vi "niRFUtil FWK Remove All Whitespaces.vi"(7 "Input String":string) -> (8 "Resultant String":string)   [LabVIEW 2015, in "niRFUtil.lvlib"]
uses:
  niRFUtil.lvlib
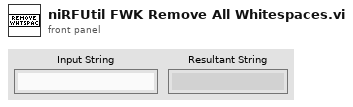
[diagram p1: front panel]
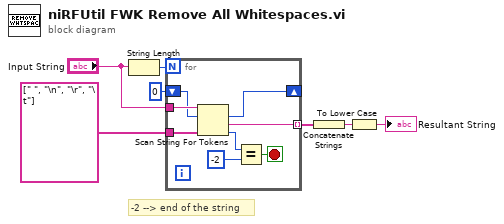
[diagram p0: block diagram]
diagram:
  # "-2 --> end of the string"
  n1 = String Length(string="Input String") -> (length=w7:i32)
  n2 = for {
    N: w7 -> [_]
    tunnel: string[] [" ", "\n", "\r", "\t"] ("Array") -> [w15]
    tunnel: "Input String" -> [w14]
    shift-right: [w8] -> _
    shift-left: 0 -> [w10]
    tunnel: [w9] -> w5 mode=indexing
    stop <- w11 stop-if-true
    n3 = Scan String For Tokens(6:w15, 8:w10, 9:w14) -> (0:w13:i32, 1:w9:string, 2:w8:i32)  [unwired: 3 in, 1 out]
    n4 = Equal?(x=w13, y=-2) -> (x = y?=w11:bool)
  }
  n5 = Concatenate Strings(w5) -> (w4:string)
  n6 = To Lower Case(string=w4) -> (all lower case string=→"Resultant String":string)
